vi "All_Combined_final.vi"() -> ()   [LabVIEW 2018]
uses:
  <vilib>/LabVIEW Interface for Arduino/Type Defs/Board Type.ctl
  Controls created/Control 3.ctl
  Controls created/Control 4.ctl
  <vilib>/LabVIEW Interface for Arduino/Type Defs/Connection Type.ctl
  <instrlib>/LeCroy Wave Series/Public/Data/Read Single Waveform.vi
  <vilib>/LabVIEW Interface for Arduino/LabVIEW Interface for Arduino.lvlib
  <instrlib>/Siglent SDG X Series/Siglent SDG X Series.lvlib
  <instrlib>/LeCroy Wave Series/LeCroy Wave Series.lvlib
panel:
  in  "Tab Control":enum32{"Page 1", "Page 2", "Page 3"}(tab)
  in  "VISA resource":refnum<visa-resource-name>
  in  "Board Type (Uno)":T1
  in  "Steps for 1 rotation(1600steps)":i16=1600
  in  "Set Speed (Steps/s)":i16=1200 min=0 max=3000 step=50
  out "Steps Remaining? 2":bool
  in  "Step Size":i16
  out "Step Angle":dbl
  in  "Baud Rate":u32=115200
  out "Iteration #":i32
  out "Steps Remaining?":bool
  in  "Total translation distance(in mm)":i16
  out "Error":errorcluster
  in  "Step size":i16
  in  "Arbitray Movement":bool
  in  "Stop":bool
  out "Moving?":bool
  out "stop motion":bool
  in  "MOTION":bool
  in  "?":i8(slide) step=2 scale=0.0..2.0
  in  "OK Button":bool
  out "# steps moved":i32
  in  "VISA Refnum in":refnum<visa-resource-name>
  in  "Channel (1:Channel 1)":i32(ring)=1 items=["Channel 1"=1, "Channel 2"=2]
  in  "Enable Output (T: Enable)":bool=TRUE
  in  "Amplitude (1.0 Vpp)":dbl=1.0 format="%#.3f"
  in  "Frequency (1000 Hz)":T2=1500000.0 format="%#.6g"
  in  "DC Offset (0.00 V) in":dbl
  in  "Waveform Function (0: Sine) in":u16(ring) items=["Sine", "Square", "Ramp", "DC", "Pulse", "Arb"]
  in  "Phase (0.0 degrees)":dbl=0.002 min=-360.0 max=360.0 format="%#.1g"
  in  "Fall (20 ns)":dbl=8.4e-09 format="%#.3g"
  in  "Duty (20%)":dbl=4.32 min=0.0001 max=100.0 format="%.4g"
  in  "Delay (0.00 s)":dbl min=-1000000.0 max=1000000.0
  in  "Rise (20 ns)":dbl=1.04e-08 format="%#.3g"
  in  "True To \ngenerate\n pulse":T3=TRUE
  out "VISA resource name out":refnum<visa-resource-name>
  out "error out":errorcluster
  out "Output Filename":path
  out "error out 2":errorcluster
  in  "format string":string="Channel: %g \nWavetype: %g \nAMP: %gV\nFreq: %gHz \nRiseTime: %gs \nFallTime: %gs \nDutyCycle: %g"
  out "Output Directory":path
  in  "File Directory":path=path "E:/Ankur/Labview/Automation/Data/Exp1"
  in  "Filename":string
  out "Oscilloscope\n Runnning":bool
  in  "stop":bool
  out "Waveform Data":waveform(dbl)(graph)
  in  "Timeout (10000 ms)":u32=10000
  in  "Source (0: Channel 1)":u16(ring) items=["Channel 1", "Channel 2", "Channel 3", "Channel 4", "Memory 1", "Memory 2", "Memory 3", "Memory 4", "Function 1", "Function 2", "Function 3", "Function 4", "Function 5", "Function 6", "Function 7", "Function 8"]
  in  "Perform Auto Setup?":bool
  in  "Reset Scope?":bool
  in  "VISA resource name":refnum<visa-resource-name>
  out "Saved filename":string
  in  "Save Files in Directory":string="D:\\Automation\\Data"
  in  "Filename":string="Title"
  # "For Rotational motion"
  # "For Translational Motion"
  # "For Translational motion"
  # "OFF"
  # "ON"
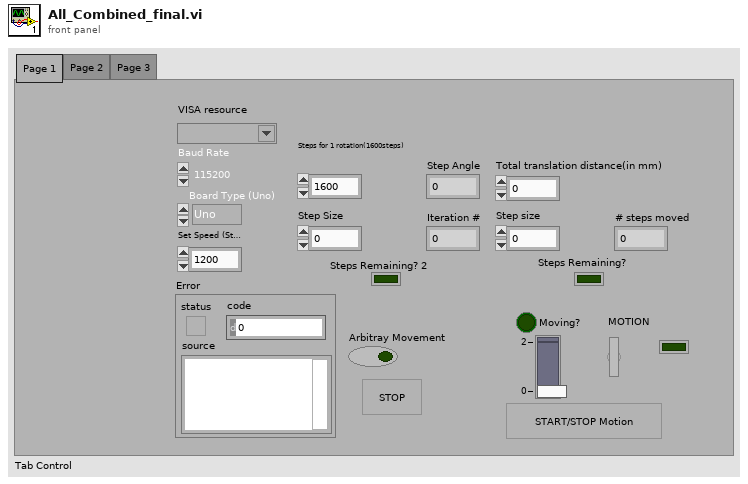
[diagram p1: front panel]
types:
  T1 = typedef "LabVIEW Interface for Arduino.lvlib/Board Type.ctl" = enum16{"Uno", "Dimuelanove w/Atmega 328", "Mega 2560"}
  T2 = typedef "Control 3.ctl" = dbl
  T3 = typedef "Control 4.ctl" = bool
  T4 = typedef "LabVIEW Interface for Arduino.lvlib/Connection Type.ctl" = enum8{"USB / Serial", "XBEE", "BlueSmirf (Bluetooth)"}
  T5 = typedef "LabVIEW Interface for Arduino.lvlib/Arduino Resource.ctl" = cluster{"VISA resource":refnum<visa-resource-name>, "Board Type":T1, "Connection Type":enum8{"USB / Serial"}, "Bytes Per Packet (15)":u8}
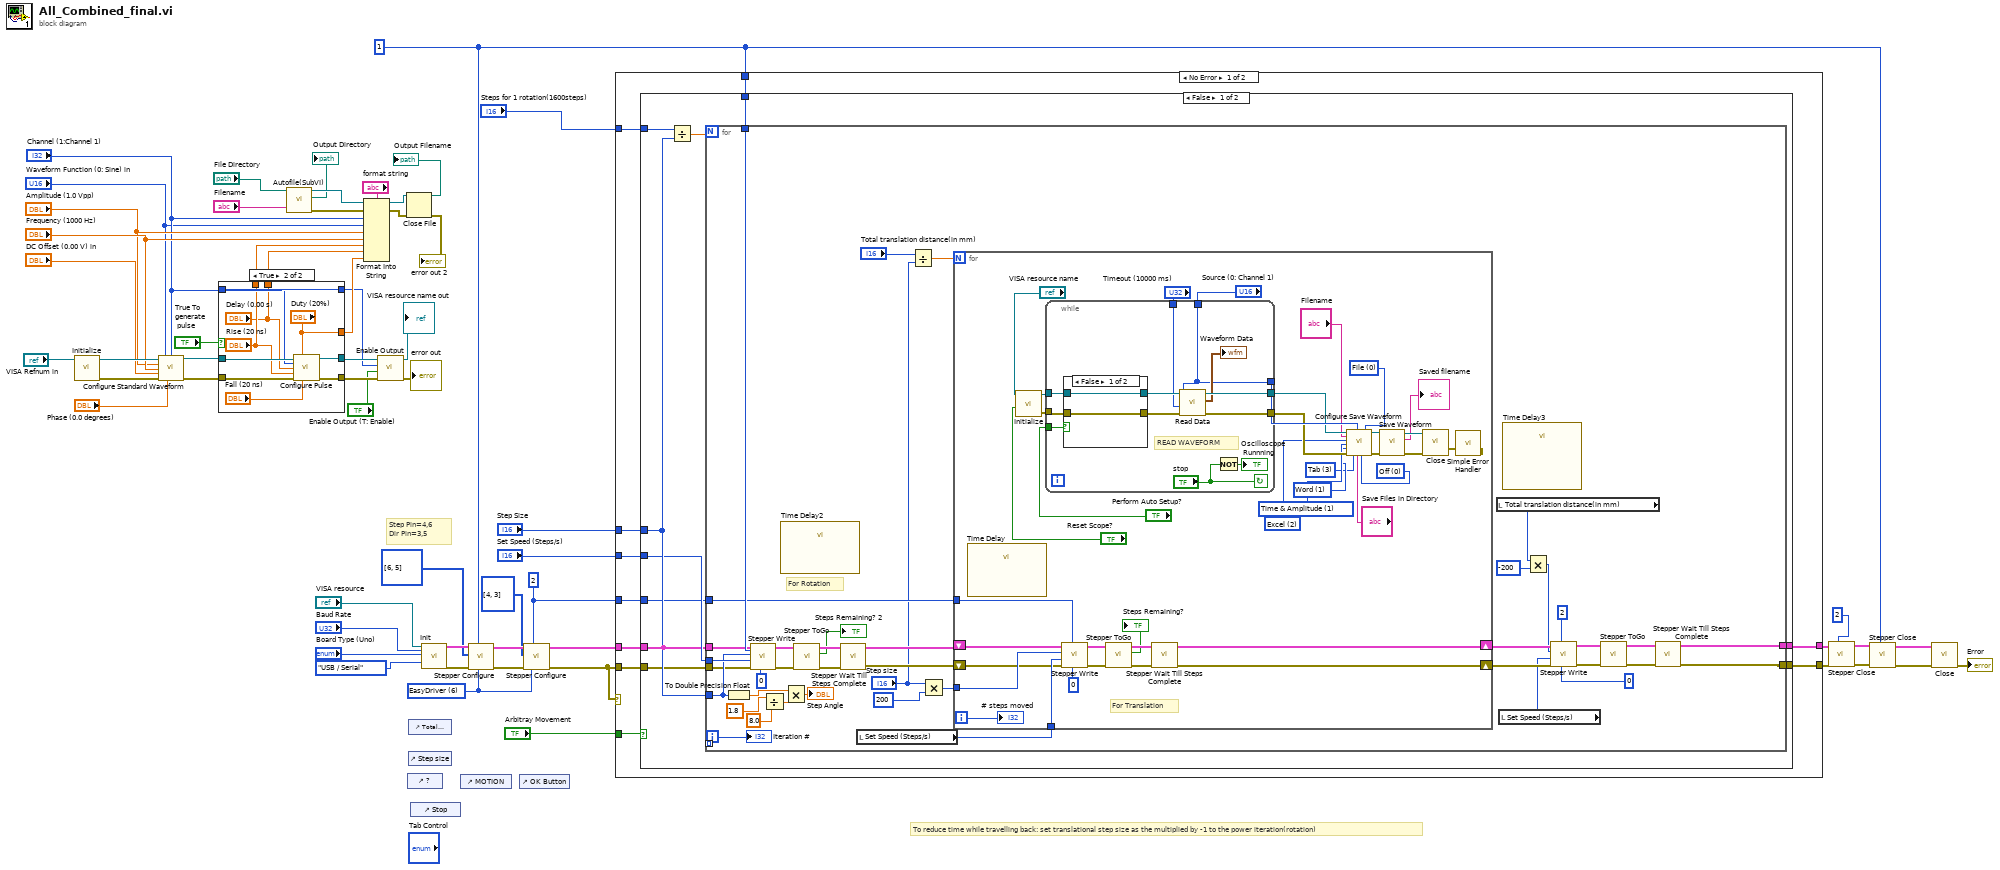
[diagram p0: block diagram]
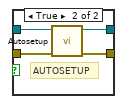
[diagram p2: hidden frame]
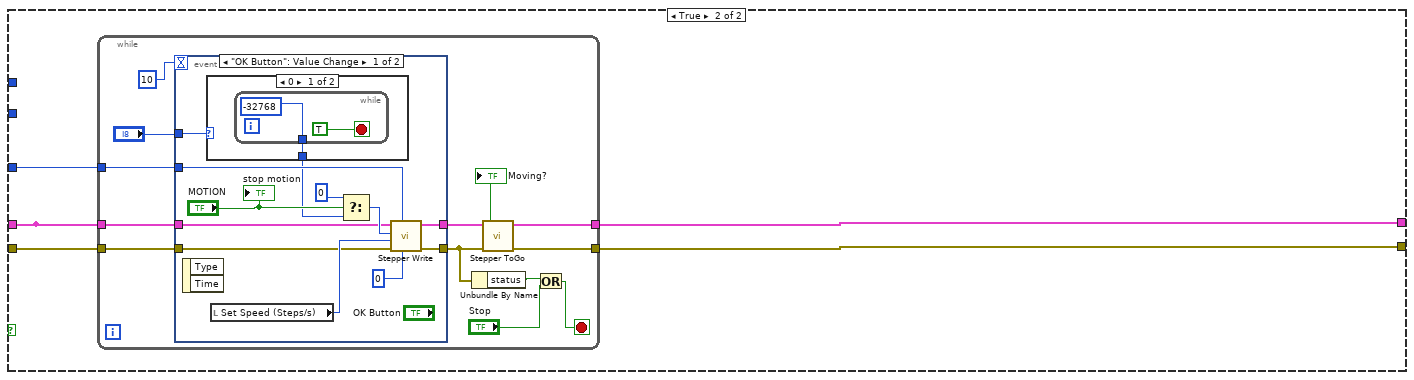
[diagram p3: hidden frame]
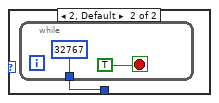
[diagram p4: hidden frame]
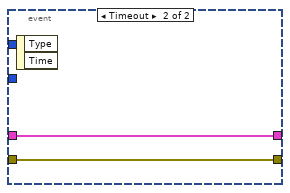
[diagram p5: hidden frame]
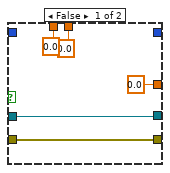
[diagram p7: hidden frame]
diagram:
  w41 = u8 2 ("Stepper #")
  w10 = u8 1 ("Stepper #")
  w42 = u8 6 items=["2 Wire (Pulse & Direction)"=1, "2 Wire"=2, "4 Wire"=4, "EasyDriver"=6, "AF Motor Shield (Stepper 1 & 2 Only)"=5] ("Control Method")
  # "To reduce time while travelling back: set translational step size as the multiplied by -1 to the power iteration(rotation)"
  # "Step Pin=4,6\nDir Pin=3,5"
  n1 = call <instrlib>:"Initialize.vi"("VISA resource name"="VISA Refnum in") -> ("error out"=w35:errorcluster, "VISA resource name out"=w36:refnum<visa-resource-name>)  [unwired: 9 in]
  n2 = call <instrlib>:"Configure Standard Waveform.vi"("VISA resource name"=w36, "Waveform Function (0: Sine)"="Waveform Function (0: Sine) in", "Channel (1:Channel 1)"="Channel (1:Channel 1)", "Amplitude (1.0 Vpp)"="Amplitude (1.0 Vpp)", "Frequency (1000 Hz)"="Frequency (1000 Hz)", "DC Offset (0.00 V)"="DC Offset (0.00 V) in", "error in (no error)"=w35, "Phase (0.0 degrees)"="Phase (0.0 degrees)") -> ("VISA resource name out"=w31:refnum<visa-resource-name>, "error out"=w34:errorcluster)  [unwired: 6 in]
  n3 = case shown="True" "True To \ngenerate\n pulse" {
    tunnel: [w62 w70] -> w40
    tunnel: [w61 w69] -> w39
    tunnel: w31 -> [w62 w68]
    tunnel: w34 -> [w61 w67]
    tunnel: "Channel (1:Channel 1)" -> [_ w66]
    tunnel: "Channel (1:Channel 1)" -> [_ _]
    tunnel: [0.0 ("Duty (20%)") "Duty (20%)"] -> w27
    tunnel: [0.0 ("Rise (20 ns)") "Rise (20 ns)"] -> w19
    tunnel: [0.0 ("Delay (0.00 s)") "Delay (0.00 s)"] -> w18
    frame False {
    }
    frame True {
      n4 = call <instrlib>:"Configure Pulse.vi"("VISA resource name"=w68, "Duty (20%)"="Duty (20%)", "Channel (1:Channel 1)"=w66, "Delay (0.00 s)"="Delay (0.00 s)", "Rise (20 ns)"="Rise (20 ns)", "error in (no error)"=w67, "Fall (20 ns)"="Fall (20 ns)") -> ("VISA resource name out"=w70:refnum<visa-resource-name>, "error out"=w69:errorcluster)  [unwired: 7 in]
    }
  }
  n5 = call "Autofile(SubVI).vi"("Filename"="Filename", "File Directory"="File Directory") -> ("error out"=w14:errorcluster, "Output Directory"=→"Output Directory":path, "Byte Stream File out"=w15:refnum<file>)  [unwired: 7 in]
  n6 = Format Into String(format string="format string", initial string=w15, error in=w14, "Channel (1:Channel 1)", "Waveform Function (0: Sine) in", "Amplitude (1.0 Vpp)", "Frequency (1000 Hz)", w19, w18, w27) -> (resulting string=w26:refnum<file>, error out=w23:errorcluster)
  n7 = call <instrlib>:"Enable Output.vi"("error in (no error)"=w39, "Enable Output (T: Enable)"="Enable Output (T: Enable)", "Channel (1:Channel 1)"="Channel (1:Channel 1)", "VISA resource name"=w40) -> ("error out"=→"error out":errorcluster, "VISA resource name out"=→"VISA resource name out":refnum<visa-resource-name>)  [unwired: 6 in]
  n8 = Close File(refnum=w26, error in=w23) -> (path=→"Output Filename":path, error out=→"error out 2":errorcluster)
  n9 = control-ref of="?"() -> ()  [unwired: 1 out]
  n10 = control-ref of="Total translation distance(in mm)"() -> ()  [unwired: 1 out]
  n11 = control-ref of="Step size"() -> ()  [unwired: 1 out]
  n12 = control-ref of="Stop"() -> ()  [unwired: 1 out]
  n13 = call <vilib>:"Init.vi"("VISA resource"="VISA resource", "Baud Rate (115200)"="Baud Rate", "Board Type (Uno)"="Board Type (Uno)", "Connection Type (USB/Serial)"=Connection_Type."USB / Serial") -> ("Arduino Resource"=w54:T5, "error out"=w53:errorcluster)  [unwired: 14 in]
  n14 = control-ref of="MOTION"() -> ()  [unwired: 1 out]
  n15 = call <vilib>:"Stepper Configure.vi"("Control Method"=w42, "Stepper #"=w10, "error in"=w53, "Stepper Pins"=u8[] [6, 5], "Arduino Resource"=w54) -> ("error out"=w44:errorcluster, "Arduino Resource Out"=w45:T5)  [unwired: 5 in]
  n16 = control-ref of="OK Button"() -> ()  [unwired: 1 out]
  n17 = call <vilib>:"Stepper Configure.vi"("Control Method"=w42, "Stepper #"=w41, "error in"=w44, "Stepper Pins"=u8[] [4, 3], "Arduino Resource"=w45) -> ("error out"=w6:errorcluster, "Arduino Resource Out"=w7:T5)  [unwired: 5 in]
  n18 = case shown="No Error" w6 {
    tunnel: [w75 w227] -> w2
    tunnel: [w82 w228] -> w1
    tunnel: [w81 w228] -> _
    tunnel: "Step Size" -> [w80 _]
    tunnel: "Steps for 1 rotation(1600steps)" -> [w79 _]
    tunnel: "Set Speed (Steps/s)" -> [w78 _]
    tunnel: "Arbitray Movement" -> [w77 _]
    tunnel: w10 -> [w76 _]
    tunnel: w41 -> [w74 _]
    tunnel: w7 -> [w73 w228]
    tunnel: w6 -> [w72 w227]
    frame No Error {
      n19 = case shown="False" w77 {
        tunnel: [w91 w193] -> w82
        tunnel: [w84 w191] -> w81
        tunnel: w80 -> [w89 _]
        tunnel: w79 -> [w88 _]
        tunnel: w78 -> [w87 _]
        tunnel: w76 -> [w86 _]
        tunnel: [w92 w189] -> w75
        tunnel: w74 -> [w85 w192]
        tunnel: w73 -> [w84 w191]
        tunnel: w72 -> [w83 w190]
        frame False {
          n20 = Divide(x=w88, y=w89) -> (x/y=w90:dbl)
          n21 = for {
            N: w90 -> [_]
            tunnel: [w98] -> w92
            tunnel: [w99] -> w91
            tunnel: w87 -> [w129]
            tunnel: [w124] -> _ mode=indexing
            tunnel: w89 -> [w123]
            tunnel: w86 -> [w118]
            tunnel: w85 -> [w117]
            tunnel: w84 -> [w108]
            tunnel: w83 -> [w107]
            i -> [w124]
            # "For Rotation"
            n22 = To Double Precision Float(number=w123) -> (double precision float=w125:dbl)
            n23 = call <vilib>:"Stepper Write.vi"("Set Acceleration (0 to disable)"=i16 0 ("Acceleration"), "Stepper #"=w118, "error in"=w107, "Set Speed (Steps per Second)"=w129, "# of Steps to Move"=w123, "Arduino Resource"=w108) -> ("error out"=w128:errorcluster, "Arduino Resource Out"=w127:T5)  [unwired: 4 in]
            n24 = Divide(x=1.8 ("y"), y=8.0) -> (x/y=w111:dbl)
            n25 = call "Time Delay2"() -> ()  [unwired: 11 in, 1 out]
            n26 = Multiply(x=w125, y=w111) -> (x*y=→"Step Angle":dbl)
            n27 = call <vilib>:"Stepper ToGo.vi"("error in"=w128, "Arduino Resource"=w127) -> ("error out"=w132:errorcluster, "Steps Remaining?"=→"Steps Remaining? 2":bool, "Arduino Resource Out"=w131:T5)  [unwired: 6 in, 1 out]
            n28 = call <vilib>:"Stepper Wait Till Steps Complete.vi"("error in"=w132, "Arduino Resource In"=w131) -> ("error out"=w122:errorcluster, "Arduino Resource Out"=w121:T5)  [unwired: 8 in]
            n29 = local read "Set Speed (Steps/s)"() -> (w120:i16)
            n30 = Divide(x="Total translation distance(in mm)", y="Step size") -> (x/y=w109:dbl)
            n31 = Multiply(x="Step size", y=i16 200) -> (x*y=w113:i16)
            n32 = for {
              N: w109 -> [_]
              shift-right: [w165] -> w101
              shift-left: w121 -> [w161]
              shift-right: [w164] -> w100
              shift-left: w122 -> [w160]
              tunnel: w113 -> [w163]
              tunnel: w120 -> [w162]
              tunnel: w117 -> [w157]
              i -> [w158]
              w135 = u16 3 items=["Comma", "Space", "Semicolon", "Tab"] ("Delimiter (  0:Comma)")
              w134 = u16 0 items=["Off", "Wrap", "Fill"] ("Auto Save (0:Off")
              w136 = u16 1 items=["Byte", "Word", "Auto"] ("BinarySubFormat (1: Word)")
              w137 = u16 1 items=["Amplitude Only", "Time & Amplitude", "With Header"] ("SubFormat (1: Time & Amplitude)")
              w138 = u16 2 items=["Binary", "ASCII", "Excel", "MATLAB", "MathCad", "WaveML"] ("Format (0: Binary)")
              w133 = u16 0 items=["File", "M1", "M2", "M3", "M4"] ("Destination (0:File)")
              # "For Translation"
              n33 = call "Time Delay"() -> ()  [unwired: 11 in, 1 out]
              n34 = call <instrlib>:"Initialize.vi"("Reset? (T: Yes)"="Reset Scope?", "VISA resource name"="VISA resource name") -> ("error out"=w143:errorcluster, "VISA resource name out"=w142:refnum<visa-resource-name>)  [unwired: 8 in]
              n35 = while {
                tunnel: [w180] -> w149
                tunnel: [w179] -> w148
                tunnel: "Perform Auto Setup?" -> [w178]
                tunnel: "Source (0: Channel 1)" -> [w171]
                tunnel: w143 -> [w177]
                tunnel: w142 -> [w176]
                tunnel: "Timeout (10000 ms)" -> [w175]
                tunnel: [w171] -> w150
                stop <- "stop" continue-if-true
                # "READ WAVEFORM"
                n36 = case shown="False" w178 {
                  tunnel: w177 -> [w183 w188]
                  tunnel: w176 -> [w184 w187]
                  tunnel: [w184 w186] -> w182
                  tunnel: [w183 w185] -> w181
                  frame False {
                  }
                  frame True {
                    # "AUTOSETUP"
                    n37 = call <instrlib>:"Autosetup.vi"("error in (no error)"=w188, "VISA resource name"=w187) -> ("error out"=w185:errorcluster, "VISA resource name out"=w186:refnum<visa-resource-name>)  [unwired: 8 in]
                  }
                }
                n38 = call-poly <instrlib>:"Read Data.vi"("error in (no error)"=w181, "Timeout (10000 ms)"=w175, "Source (0: Channel 1)"=w171, "VISA resource name"=w182) -> ("error out"=w180:errorcluster, "Waveform Data"=→"Waveform Data":waveform(dbl), "VISA resource name out"=w179:refnum<visa-resource-name>)  [unwired: 5 in]
                n39 = Not(x="stop") -> (.not. x?=→"Oscilloscope\n Runnning":bool)
              }
              n40 = call <vilib>:"Stepper Write.vi"("Set Acceleration (0 to disable)"=i16 0, "Stepper #"=w157, "error in"=w160, "Set Speed (Steps per Second)"=w162, "# of Steps to Move"=w163, "Arduino Resource"=w161) -> ("error out"=w167:errorcluster, "Arduino Resource Out"=w166:T5)  [unwired: 4 in]
              n41 = call <vilib>:"Stepper ToGo.vi"("error in"=w167, "Arduino Resource"=w166) -> ("error out"=w170:errorcluster, "Steps Remaining?"=→"Steps Remaining?":bool, "Arduino Resource Out"=w169:T5)  [unwired: 6 in, 1 out]
              n42 = call <vilib>:"Stepper Wait Till Steps Complete.vi"("error in"=w170, "Arduino Resource In"=w169) -> ("error out"=w164:errorcluster, "Arduino Resource Out"=w165:T5)  [unwired: 8 in]
              n43 = call <instrlib>:"Configure Save Waveform.vi"("VISA resource name"=w148, "Trace Title (Title)"="Filename", "Format (0: Binary)"=w138, "SubFormat (1: Time & Amplitude)"=w137, "BinarySubFormat (1: Word)"=w136, "error in (no error)"=w149, "Delimiter (  0:Comma)"=w135, "Source (0: Channel 1)"=w150, "Save Files in Directory (D:\\Waveforms)"="Save Files in Directory", "Auto Save (0:Off"=w134, "Destination (0:File)"=w133) -> ("VISA resource name out"=w152:refnum<visa-resource-name>, "error out"=w153:errorcluster)  [unwired: 7 in]
              n44 = call <instrlib>:"Save Waveform.vi"("error in (no error)"=w153, "VISA resource name"=w152) -> ("error out"=w156:errorcluster, "Saved filename"=→"Saved filename":string, "VISA resource name out"=w155:refnum<visa-resource-name>)  [unwired: 7 in]
              n45 = call <vilib>:"Close.vi"("error in (no error)"=w156, "VISA resource name"=w155) -> ("error out"=w140:errorcluster)  [unwired: 9 in]
              n46 = call <vilib>:"Simple Error Handler.vi"("error in (no error)"=w140) -> ()  [unwired: 4 in, 5 out]
              "# steps moved" <- w158
            }
            n47 = local read "Total translation distance(in mm)"() -> (w96:i16)
            n48 = local read "Set Speed (Steps/s)"() -> (w93:i16)
            n49 = call "Time Delay3"() -> ()  [unwired: 11 in, 1 out]
            n50 = Multiply(x=w96, y=i16 -200) -> (x*y=w94:i16)
            n51 = call <vilib>:"Stepper Write.vi"("Set Acceleration (0 to disable)"=i16 0, "Stepper #"=u8 2, "error in"=w100, "Set Speed (Steps per Second)"=w93, "# of Steps to Move"=w94, "Arduino Resource"=w101) -> ("error out"=w104:errorcluster, "Arduino Resource Out"=w103:T5)  [unwired: 4 in]
            n52 = call <vilib>:"Stepper ToGo.vi"("error in"=w104, "Arduino Resource"=w103) -> ("error out"=w106:errorcluster, "Arduino Resource Out"=w105:T5)  [unwired: 6 in, 2 out]
            n53 = call <vilib>:"Stepper Wait Till Steps Complete.vi"("error in"=w106, "Arduino Resource In"=w105) -> ("error out"=w98:errorcluster, "Arduino Resource Out"=w99:T5)  [unwired: 8 in]
            "Iteration #" <- w124
          }
        }
        frame True {
          n54 = while {
            tunnel: [w199] -> w193
            tunnel: w192 -> [w198]
            tunnel: w191 -> [w196]
            tunnel: w190 -> [w195]
            tunnel: [w194] -> w189
            stop <- w205 stop-if-true
            n55 = event shown="[0] \"OK Button\": Value Change" {
              selector: _ -> [_ _]
              dyn-events: _ -> [_ _]
              timeout: 10 -> [_ _]
              tunnel: [w217 w226] -> w203
              tunnel: [w218 w225] -> w201
              tunnel: w198 -> [w213 _]
              tunnel: "?" -> [w211 _]
              tunnel: w196 -> [w208 w226]
              tunnel: w195 -> [w207 w225]
              event "OK Button": Value Change {
                n56 = event-data() -> ()  [unwired: 1 in, 2 out]
                n57 = case shown="0" w211 {
                  tunnel: [w219 w222] -> w209
                  frame 0 {
                    n58 = while {
                      tunnel: [i16 -32768 ("# of Steps to Move")] -> w219
                      stop <- TRUE ("Stop Reverse movement") stop-if-true
                    }
                  }
                  frame 2, Default {
                    n59 = while {
                      tunnel: [i16 32767 ("# of Steps to Move")] -> w222
                      stop <- TRUE ("Stop Forward movement") stop-if-true
                    }
                  }
                }
                n60 = local read "Set Speed (Steps/s)"() -> (w212:i16)
                n61 = Select(t=0, s="MOTION", f=w209) -> (s? t:f=w214:i32)
                n62 = call <vilib>:"Stepper Write.vi"("Set Acceleration (0 to disable)"=i16 0 ("Set acceleration"), "Stepper #"=w213, "error in"=w207, "Set Speed (Steps per Second)"=w212, "# of Steps to Move"=w214, "Arduino Resource"=w208) -> ("error out"=w218:errorcluster, "Arduino Resource Out"=w217:T5)  [unwired: 4 in]
                "stop motion" <- "MOTION"
              }
              event Timeout {
                n63 = event-data() -> ()  [unwired: 1 in, 2 out]
              }
            }
            n64 = Unbundle By Name(w201) -> ("status"=w204:bool)
            n65 = call <vilib>:"Stepper ToGo.vi"("error in"=w201, "Arduino Resource"=w203) -> ("error out"=w194:errorcluster, "Steps Remaining?"=→"Moving?":bool, "Arduino Resource Out"=w199:T5)  [unwired: 6 in, 1 out]
            n66 = Or(x=w204, y="Stop") -> (x .or. y?=w205:bool)
          }
        }
      }
    }
    frame Error {
    }
  }
  n67 = call <vilib>:"Stepper Close.vi"("Stepper #"=u8 2, "error in"=w2, "Arduino Resource"=w1) -> ("error out"=w5:errorcluster, "Arduino Resource Out"=w4:T5)  [unwired: 7 in]
  n68 = call <vilib>:"Stepper Close.vi"("Stepper #"=w10, "error in"=w5, "Arduino Resource"=w4) -> ("error out"=w9:errorcluster, "Arduino Resource Out"=w8:T5)  [unwired: 7 in]
  n69 = call <vilib>:"Close.vi"("Arduino Resource"=w8, "error in"=w9) -> ("error out"=→"Error":errorcluster)  [unwired: 13 in]
